vi "Vision Processing.vi"(4 "error in (no error)":errorcluster, 5 "Camera Type":enum16{"206", "1011"}(ring)=enum."1011", 6 "Input Image":T1, 7 "Enable Vision":bool) -> (2 "Processed Image":T1(plugin-control))   [LabVIEW 2011]
uses:
  <vilib>/vision/Image Controls.llb/IMAQ Image.ctl
  Robot Global Data.vi
  <vilib>/vision/NI_Vision_Development_Module.lvlib
panel:
  out "Target Info":T2(array[cluster])
  in  "Area Size Limit":i32=444
  in  "Particle Count Limit":i32=8
  in  "Score Limits":T3={"Rect Coverage"=76.0, "Aspect Ratio"=70.0, "X Edge Strength"=40.0, "Y Edge Strength"=60.0}
  in  "Processing":enum32{"Color", "Intensity", "Intensity Open"}(tab)
  in  "Luminance":i32=255
  in  "Saturation":i32=255
  in  "Hue":i32(knob)=65 scale=0.0..255.0
  in  "Margins":cluster{"Hue":i32, "Sat":i32, "Lum":i32}={"Hue"=20, "Sat"=27, "Lum"=30} {"Sat" scale=0.0..40.0; "Lum" scale=0.0..40.0; "Hue" scale=0.0..40.0}
  in  "Range":cluster{"Lower value":sgl, "Upper value":sgl}={"Lower value"=150.0, "Upper value"=255.0} {"Lower value" scale=0.0..255.0; "Upper value" scale=0.0..255.0}
  in  "Range":cluster{"Lower value":sgl, "Upper value":sgl}={"Lower value"=150.0, "Upper value"=255.0} {"Lower value" scale=0.0..255.0; "Upper value" scale=0.0..255.0}
  out "Original Image":T1(plugin-control)
  # "Instructions:\nProcessing the reflective tape that is illuminated by a ring light can be based\non color or light intensity.\nParticles within the image are scored by rectangle coverage, aspect ratio, and\nfor being hollow with a bold edge. A particle is considered a target if all scores\nare above the score limits. Particles can be annotated -- surrounded by\na rectangle and scores drawn to the left .\nTo control the number of particles being scored, use the count limit and the size\nlimit."
  # "To debug, Enable using the View button.\nFor color processing, you can click in the image to select the color for processing."
  # "Enable by clicking the View button.\nGreen scores are above the limit, orange are below. Inner/outer rect\nindicates all passed."
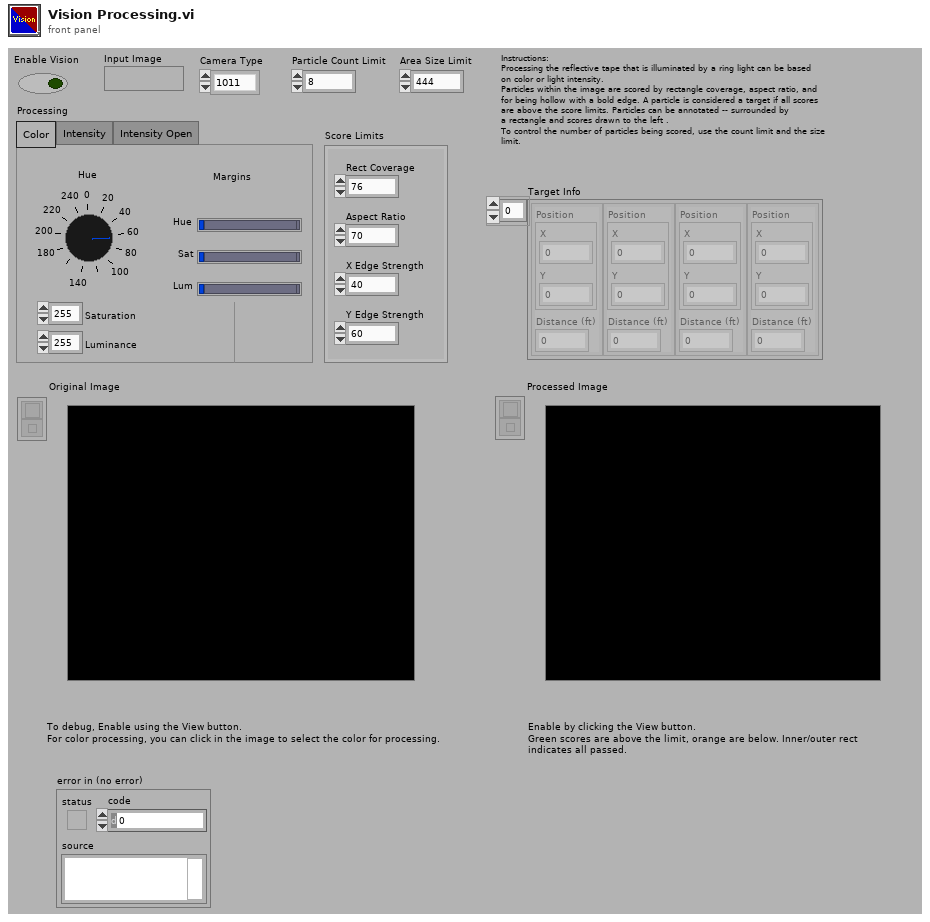
[diagram p1: front panel]
types:
  T1 = typedef "IMAQ Image.ctl" = refnum<image>
  T2 = cluster{"Position":cluster{"X":dbl, "Y":dbl}, "Distance (ft)":dbl}[]
  T3 = cluster{"Rect Coverage":dbl, "Aspect Ratio":dbl, "X Edge Strength":dbl, "Y Edge Strength":dbl}
  T4 = typedef "Image Type" = u32
  T5 = typedef "WPI_CameraImageSize.ctl" = enum16{"640x480", "320x240", "160x120"}
  T6 = enum32{"AutoM", "Close", "Dilate", "Erode", "Gradient", "Gradient out", "Gradient in", "Hit miss", "Open", "PClose", "POpen", "Thick", "Thin"}
  T7 = cluster{cluster{"Left":dbl, "Top":dbl, "Right":dbl, "Bottom":dbl}, dbl[]}[]
  T8 = cluster{"Left":dbl, "Top":dbl, "Right":dbl, "Bottom":dbl}
  T9 = cluster{"Target Center (-1 to 1)":cluster{"X":dbl, "Y":dbl}, "Distance (ft)":dbl}
  T10 = cluster{"Target Center (-1 to 1)":cluster{"X":dbl, "Y":dbl}, "Distance (ft)":dbl}[]
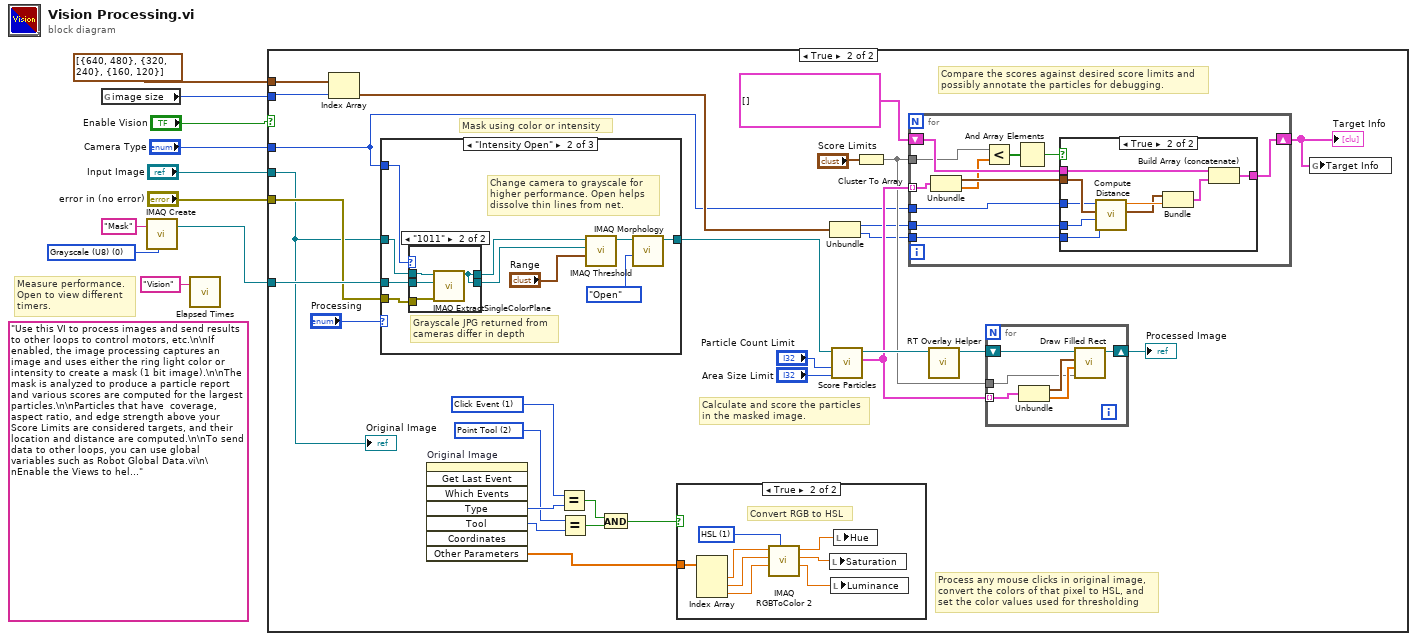
[diagram p0: block diagram]
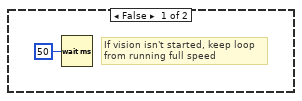
[diagram p2: hidden frame]
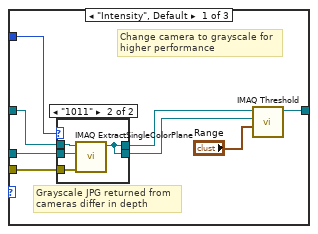
[diagram p4: hidden frame]
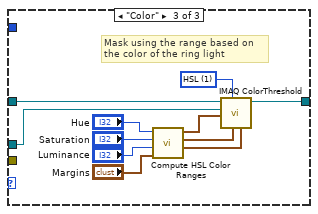
[diagram p7: hidden frame]
diagram:
  w10 = T4 0 items=["Grayscale (U8)", "Grayscale (I16)", "Grayscale (SGL)", "Complex (CSG)", "RGB (U32)", "HSL (U32)", "RGB (U64)", "Grayscale (U16)"] ("Image Type")
  (unwired) "Use this VI to process images and send results to other loops to control motors, etc.\n\nIf enabled, the image processing captures an image and uses either the ring light color or intensity to create a mask (1 bit image).\n\nThe mask is analyzed to produce a particle report and various scores are computed for the largest particles.\n\nParticles that have  coverage, aspect ratio, and edge strength above your Score Limits are considered targets, and their location and distance are computed.\n\nTo send data to other loops, you can use global variables such as Robot Global Data.vi\n\nEnable the Views to help debug color settings. Disable the View to speed up processing."
  # "Measure performance.\nOpen to view different\ntimers."
  n1 = global read "Robot Global Data.vi" "image size"() -> (w6:T5)
  n2 = call "IMAQ Create"("Image Name"="Mask", "Image Type"=w10) -> ("New Image"=w1:T1)  [unwired: 2 in, 2 out]
  n3 = call "Elapsed Times.vi"("Call Name"="Vision") -> ()  [unwired: 2 in, 1 out]
  n4 = case shown="True" "Enable Vision" {
    tunnel: "Input Image" -> [_ w21]
    tunnel: w6 -> [_ w28]
    tunnel: w1 -> [_ w23]
    tunnel: cluster{i32, i32}[] [{640, 480}, {320, 240}, {160, 120}] -> [_ w27]
    tunnel: "error in (no error)" -> [_ w22]
    tunnel: "Camera Type" -> [_ w12]
    frame False {
      # "If vision isn't started, keep loop\nfrom running full speed"
      n5 = Wait (ms)(milliseconds to wait=u32 50) -> ()  [unwired: 1 out]
    }
    frame True {
      w15 = 2 items=["None", "Selection Tool", "Point Tool", "Line Tool", "Rectangle Tool", "Oval Tool", "Polygon Tool", "ClosedFreehandTool", "Annulus Tool", "Rotated Rectangle Tool", "Zoom Tool", "Pan Tool", "Polyline Tool", "Freehand Tool"] ("Tool")
      w16 = 1 items=["No Event"=0, "Click Event"=1, "Draw Event"=2, "Size Event"=4, "Scroll Event"=5, "Double Click Event"=8] ("Type")
      # "Compare the scores against desired score limits and\npossibly annotate the particles for debugging."
      # "Process any mouse clicks in original image,\nconvert the colors of that pixel to HSL, and\nset the color values used for thresholding"
      # "Calculate and score the particles\nin the masked image."
      # "Mask using color or intensity"
      n6 = Index Array(array=w27, index=w28) -> (element=w24:cluster{i32, i32})
      n7 = case shown="\"Intensity Open\"" "Processing" {
        tunnel: [w61 w75 w95] -> w31
        tunnel: w23 -> [w60 w73 w86]
        tunnel: w12 -> [w59 w74 _]
        tunnel: w22 -> [w55 w69 _]
        tunnel: w21 -> [w56 w70 w85]
        frame "Intensity", Default {
          # "Grayscale JPG returned from\ncameras differ in depth"
          # "Change camera to grayscale for\nhigher performance"
          n8 = case shown="\"1011\"" w59 {
            tunnel: w60 -> [w64 w68]
            tunnel: [w63 w67] -> w58
            tunnel: [w64 w67] -> w57
            tunnel: w56 -> [w63 w66]
            tunnel: w55 -> [_ w65]
            frame "206", Default {
            }
            frame "1011" {
              n9 = call "IMAQ ExtractSingleColorPlane"("error in (no error)"=w65, "Image Dst"=w68, "Image Src"=w66) -> ("Image Dst Out"=w67:T1)  [unwired: 7 in, 1 out]
            }
          }
          n10 = call "IMAQ Threshold"("Range"="Range", "Image Dst"=w57, "Image Src"=w58) -> ("Image Dst Out"=w61:T1)  [unwired: 3 in, 5 out]
        }
        frame "Intensity Open" {
          # "Grayscale JPG returned from\ncameras differ in depth"
          # "Change camera to grayscale for\nhigher performance. Open helps\ndissolve thin lines from net."
          n11 = case shown="\"1011\"" w74 {
            tunnel: w73 -> [w80 w83]
            tunnel: [w79 w84] -> w72
            tunnel: [w80 w84] -> w71
            tunnel: w70 -> [w79 w82]
            tunnel: w69 -> [_ w81]
            frame "206", Default {
            }
            frame "1011" {
              n12 = call "IMAQ ExtractSingleColorPlane"("error in (no error)"=w81, "Image Dst"=w83, "Image Src"=w82) -> ("Image Dst Out"=w84:T1)  [unwired: 7 in, 1 out]
            }
          }
          n13 = call "IMAQ Threshold"("Range"="Range", "Image Dst"=w71, "Image Src"=w72) -> ("Image Dst Out"=w76:T1)  [unwired: 3 in, 5 out]
          n14 = call "IMAQ Morphology"("Operation"=T6."Open", "Image Src"=w76) -> ("Image Dst Out"=w75:T1)  [unwired: 8 in, 1 out]
        }
        frame "Color" {
          w94 = u16 1 items=["RGB", "HSL", "HSV", "HSI"] ("Color Mode")
          # "Mask using the range based on\nthe color of the ring light"
          n15 = call "Compute HSL Color Ranges.vi"("Margins"="Margins", "Luminance"="Luminance", "Saturation"="Saturation", "Hue"="Hue") -> ("Lum Range"=w91:cluster{i32, i32}, "Sat Range"=w92:cluster{i32, i32}, "Hue Range"=w93:cluster{i32, i32})  [unwired: 5 in]
          n16 = call "IMAQ ColorThreshold"("Blue or Luma or Val or Inten Range"=w91, "Green or Sat Range"=w92, "Color Mode"=w94, "Red or Hue Range"=w93, "Image Dst"=w86, "Image Src"=w85) -> ("Image Dst Out"=w95:T1)  [unwired: 4 in, 1 out]
        }
      }
      n17 = invoke on="Original Image" class="ImageControl" method="Get Last Event"() -> ("Type"=w17:i32, "Tool"=w20:i32, "Other Parameters"=w29:sgl[])  [unwired: 8 in, 5 out]
      n18 = Equal?(x=w16, y=w17) -> (x = y?=w18:bool)
      n19 = Equal?(x=w15, y=w20) -> (x = y?=w19:bool)
      n20 = And(x=w18, y=w19) -> (x .and. y?=w30:bool)
      n21 = case shown="True" w30 {
        tunnel: w29 -> [_ w54]
        frame False {
        }
        frame True {
          w53 = u16 1 items=["RGB", "HSL", "HSV", "HSI", "CIE L*a*b*", "CIE XYZ"] ("Color Mode")
          # "Convert RGB to HSL"
          n22 = Index Array(array=w54) -> (element #1=w52:sgl, element #2=w50:sgl, element #3=w48:sgl)  [unwired: 3 in]
          n23 = call "IMAQ RGBToColor 2"("Color Mode"=w53, "Blue value"=w48, "Green value"=w50, "Red value"=w52) -> ("Blue or Luma or Val or Inten or Z or b*value"=w47:dbl, "Green or Sat or Y or a* value"=w49:dbl, "Red or Hue or X or L* value"=w51:dbl)  [unwired: 4 in, 1 out]
          n24 = local write "Saturation"(w49) -> ()
          n25 = local write "Luminance"(w47) -> ()
          n26 = local write "Hue"(w51) -> ()
        }
      }
      n27 = Unbundle(w24) -> (w26:i32, w25:i32)
      n28 = call "Score Particles.vi"("Area Size Limit"="Area Size Limit", "Particle Count Limit"="Particle Count Limit", "Image Refnum in"=w31) -> ("Scored Particle Info"=w36:T7, "Image Refnum out"=w39:T1)  [unwired: 7 in]
      n29 = Cluster To Array(cluster="Score Limits") -> (array=w35:dbl[])
      n30 = for {
        shift-right: [w105] -> w32
        shift-left: T2 [] -> [w106]
        tunnel: w26 -> [w104]
        tunnel: w36 -> [w102] mode=indexing
        tunnel: w35 -> [w97]
        tunnel: w12 -> [w101]
        tunnel: w25 -> [w96]
        n31 = Unbundle(w102) -> (w103:T8, w98:dbl[])
        n32 = Less?(x=w97, y=w98) -> (x < y?=w100:bool[])
        n33 = And Array Elements(Boolean array=w100) -> (logical AND=w99:bool)
        n34 = case shown="True" w99 {
          tunnel: w106 -> [w107 w116]
          tunnel: [w107 w115] -> w105
          tunnel: w103 -> [_ w111]
          tunnel: w104 -> [_ w113]
          tunnel: w101 -> [_ w110]
          tunnel: w96 -> [_ w109]
          frame False {
          }
          frame True {
            n35 = call "Compute Distance.vi"("Y Image Resolution"=w109, "X Image Resolution"=w113, "Bounding Box"=w111, "Camera Type"=w110) -> ("Target Center (-1 to 1)"=w108:cluster{"X":dbl, "Y":dbl}, "Distance (ft)"=w112:dbl)  [unwired: 6 in]
            n36 = Bundle("Target Center (-1 to 1)"=w108, "Distance (ft)"=w112) -> (w114:T9)  [unwired: 1 in]
            n37 = Build Array (concatenate)(w116, w114) -> (w115:T10)
          }
        }
      }
      "Target Info" <- w32
      n38 = call "RT Overlay Helper.vi"("Refnum in"=w39) -> ("Refnum out"=w14:T1)  [unwired: 10 in]
      n39 = for {
        shift-right: [w45] -> w13
        shift-left: w14 -> [w46]
        tunnel: w36 -> [w42] mode=indexing
        tunnel: w35 -> [w41]
        n40 = Unbundle(w42) -> (w43:T8, w44:dbl[])
        n41 = call "Draw Filled Rect.vi"("Limits"=w41, "Scores"=w44, "Bounding Box"=w43, "image in"=w46) -> ("image out"=w45:T1)  [unwired: 7 in]
      }
      "Processed Image" <- w13
      n42 = global write "Robot Global Data.vi" "Target Info"(w32) -> ()
      "Original Image" <- w21
    }
  }
